vi "F8588A set & read standalone.vi"() -> ()   [LabVIEW 2020]
uses:
  0877c1e3-cff1-4e1c-ae5b-e7c7f4b59a18.vi
  eb5dc96a-a43c-4ad0-98b0-8bae309643aa.vi
  <vilib>/Analysis/NI_AALBase.lvlib
panel:
  out "time to read data (ms)":u32
  out "type A uncertainty":dbl format="%.9pV"
  out "samples":i32
  out "standard deviation":dbl format="%.9pV"
  out "mean":dbl format="%.9pV"
  in  "Initialization configuration":string="*CLS\n*RST\nDISP ON;\n*CLS\nFUNC \"DIG:VOLT\";DIG:VOLT:RANG 10.000000;\nDIG:FILT OFF;:SENS:DIG:VOLT:COUP:SIGN DCAuto;:TRIG:RESET;:TRIG:ECO 1;:ARM:LAY2:SOUR IMM;:ARM:LAY2:COUNT 1;:ARM:LAY1:COUNT 1;:ARM:LAY2:ECO 1;:ARM:LAY1:ECO 1;:ROUT:TOUT APE;:ROUT:INP:GUARD 0\nDIG:VOLT:RANG 10.000000;\n:ARM:LAY2:SOUR IMM;:ARM:LAY1:SOUR IMM;:TRIG:COUNT 101010;:TRIG:SOUR TIMER;\n:TRIG:TIMER 200E-9;\n:SENS:DIG:APER 200E-9;\nFORM PACK,2;FORM:BORD SWAP;\n:ARM:LAY1:SLOP POS;:ARM:LAY1:LEV 0.00000;:ARM:LAY1:COUP DC;\n:ARM:LAY1:DEL 1.000000E-7;\nROUT:TOUT APE;\n*CLS;"
  out "XY Graph":cluster{dbl[], dbl[]}(graph)
  out "form scale":dbl
  out "error 1":errorcluster
  out "buffer length":i32
  out "FORM?":string
  out "error 2":errorcluster
  out "read buffer":string
  # "Basic IV to test errors of F8588 communications"
  # "ASC\ndata:\n+8.407E-2\n+9.497E-2\ndecimal dot, new line as line feed (\\n),\n\nPACK,4\ndata:\nAD30 AAFF 0000 0000 8C5F 99FF 0000 0000 90E8 88FF 0000 0000\nreshape every 2nd, keep length 1, I32 little endian\n\nPACK,2\ndata:\n6CFE 2000 0000 0000 74FE 2000 0000 0000 \nreshape every 4th, keep length 1, I16 little endian\n\nPACK - nefunguje"
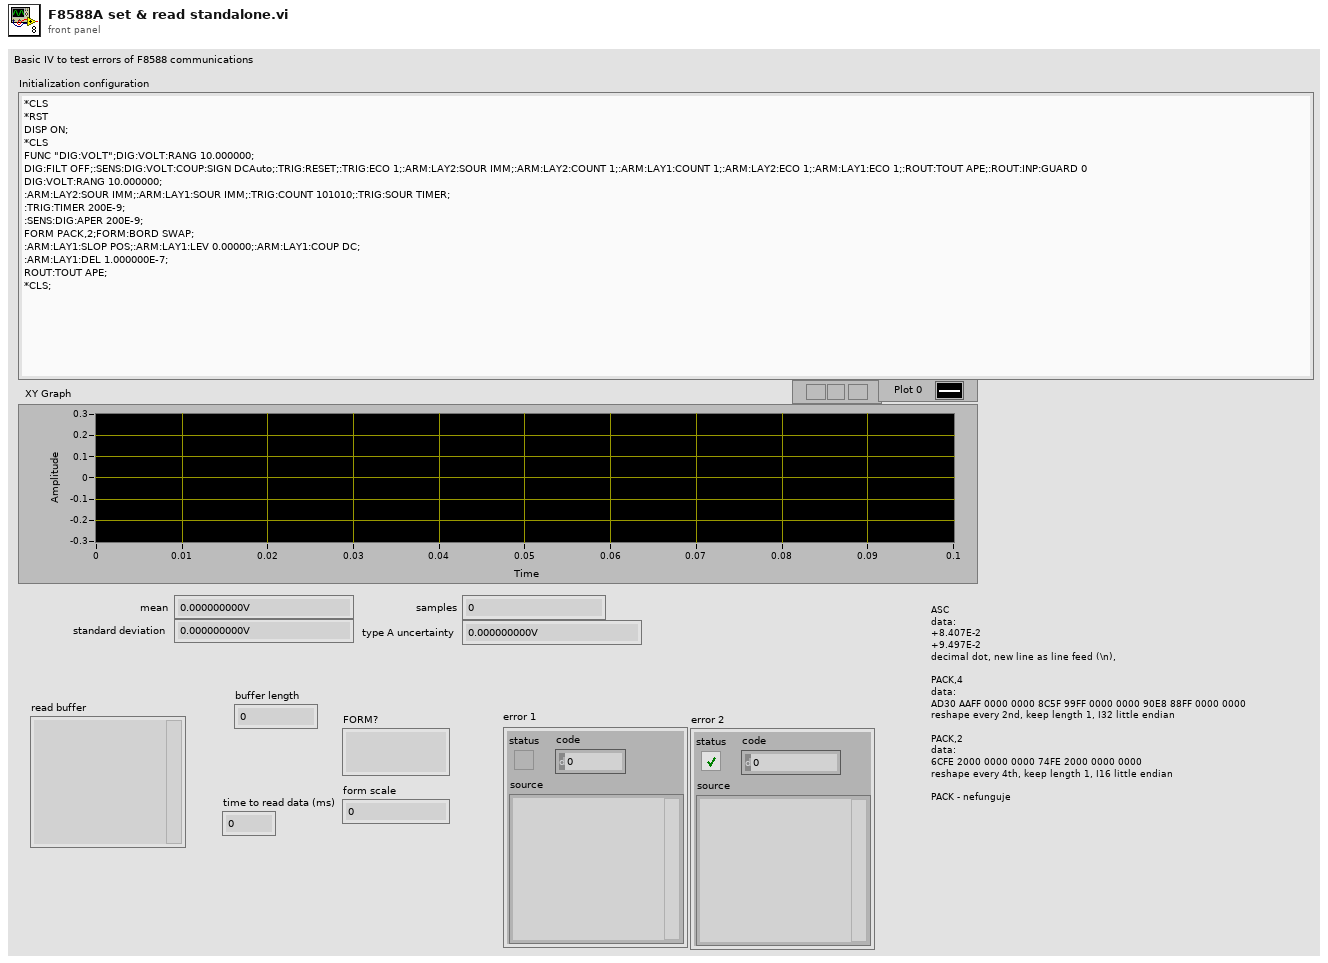
[diagram p1: front panel]
types:
  T1 = enum16{"big-endian, network order", "native, host order", "little-endian"}
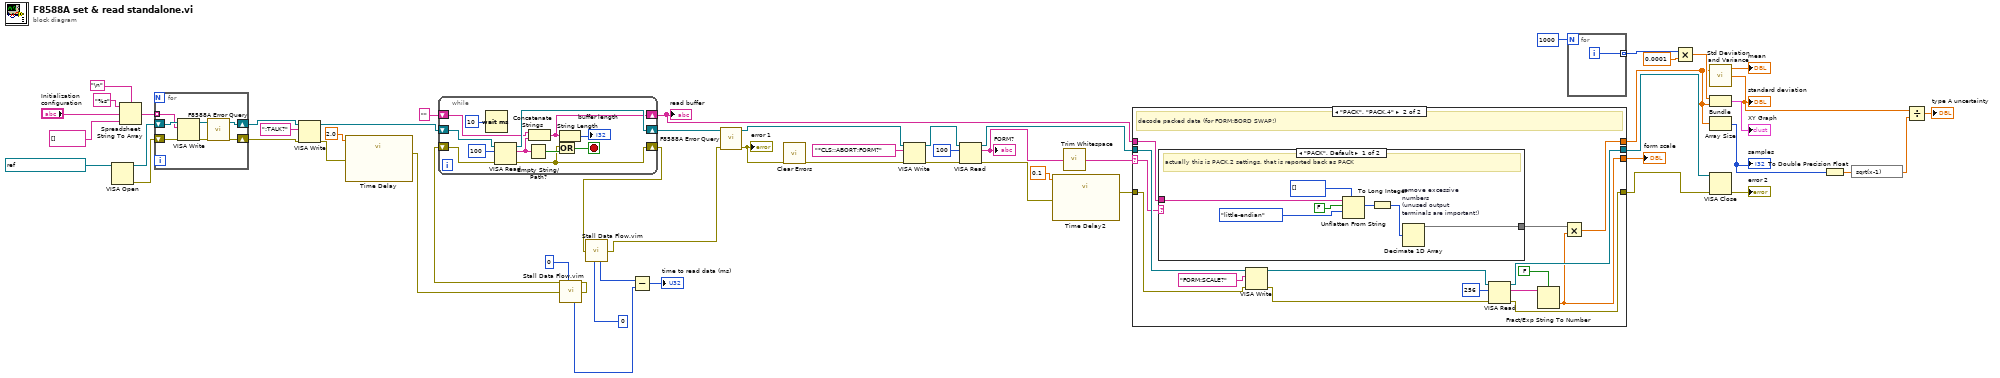
[diagram p0: block diagram]
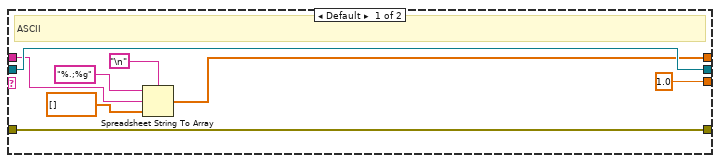
[diagram p2: hidden frame]
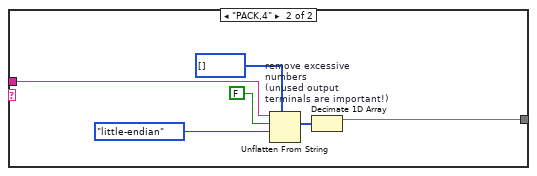
[diagram p3: hidden frame]
diagram:
  n1 = VISA Open(VISA resource name=refnum<visa-resource-name> "GPIB0::10::INSTR") -> (VISA resource name=w51:refnum<visa-resource-name>, error out=w52:errorcluster)  [unwired: 4 in]
  n2 = Spreadsheet String To Array(delimiter (Tab)="\n", format string="%s", spreadsheet string="Initialization configuration", array type (2D Dbl)=string[] []) -> (array=w46:string[])
  n3 = for {
    tunnel: w46 -> [w60] mode=indexing
    shift-right: [w58] -> w37
    shift-left: w52 -> [w62]
    shift-right: [w57] -> w38
    shift-left: w51 -> [w61]
    n4 = VISA Write(VISA resource name=w61, write buffer=w60, error in (no error)=w62) -> (VISA resource name out=w56:refnum<visa-resource-name>, error out=w59:errorcluster)  [unwired: 1 out]
    n5 = call "F8588A Error Query.vi"("error in (no error)"=w59, "VISA resource name"=w56) -> ("error out"=w58:errorcluster, "VISA resource name out"=w57:refnum<visa-resource-name>)  [unwired: 6 in, 2 out]
  }
  n6 = VISA Write(VISA resource name=w38, write buffer=":TALK?", error in (no error)=w37) -> (VISA resource name out=w35:refnum<visa-resource-name>, error out=w36:errorcluster)  [unwired: 1 out]
  n7 = call "Time Delay"("error in (no error)"=w36, "Delay Time (s)"=2.0) -> ("error out"=w4:errorcluster)  [unwired: 9 in]
  n8 = call "Stall Data Flow.vim"("value in"=w4, "milliseconds to wait"=u32 0) -> ("millisecond timer value"=w8:u32, "value out"=w3:errorcluster)
  n9 = while {
    shift-right: [w67] -> w2
    shift-left: w3 -> [w73]
    shift-right: [w72] -> w40
    shift-left: w35 -> [w71]
    shift-right: [w64] -> w25
    shift-left: "" -> [w63]
    stop <- w68 stop-if-true
    n10 = Wait (ms)(milliseconds to wait=u32 10) -> ()  [unwired: 1 out]
    n11 = VISA Read(VISA resource name=w71, byte count=u32 100, error in (no error)=w73) -> (VISA resource name out=w72:refnum<visa-resource-name>, read buffer=w70:string, error out=w67:errorcluster)  [unwired: 1 out]
    n12 = Empty String/Path?(string/path=w70) -> (empty?=w69:bool)
    n13 = Concatenate Strings(w63, w70) -> (w64:string)
    n14 = Or(x=w67, y=w69) -> (x .or. y?=w68:bool)
    n15 = String Length(string=w64) -> (length=→"buffer length":i32)
  }
  "read buffer" <- w25
  n16 = call "Stall Data Flow.vim"("value in"=w2, "milliseconds to wait"=u32 0) -> ("millisecond timer value"=w9:u32, "value out"=w1:errorcluster)
  n17 = Subtract(x=w9, y=w8) -> (x-y=→"time to read data (ms)":u32)
  n18 = call "F8588A Error Query.vi"("error in (no error)"=w1, "VISA resource name"=w40) -> ("error out"=w33:errorcluster, "VISA resource name out"=w39:refnum<visa-resource-name>)  [unwired: 6 in, 2 out]
  "error 1" <- w33
  n19 = call <vilib>:"Clear Errors.vi"("error in (no error)"=w33) -> ("error out"=w32:errorcluster)  [unwired: 5 in, 1 out]
  n20 = VISA Write(VISA resource name=w39, write buffer="*CLS;:ABORT;FORM?", error in (no error)=w32) -> (VISA resource name out=w44:refnum<visa-resource-name>, error out=w45:errorcluster)  [unwired: 1 out]
  n21 = VISA Read(VISA resource name=w44, byte count=u32 100, error in (no error)=w45) -> (VISA resource name out=w29:refnum<visa-resource-name>, read buffer=w27:string, error out=w42:errorcluster)  [unwired: 1 out]
  "FORM?" <- w27
  n22 = call "Time Delay2"("error in (no error)"=w42, "Delay Time (s)"=0.1) -> ("error out"=w6:errorcluster)  [unwired: 9 in]
  n23 = call <vilib>:"Trim Whitespace.vi"("string"=w27) -> ("trimmed string"=w26:string)  [unwired: 1 in]
  n24 = case shown="\"PACK\", \"PACK,4\"" w26 {
    selector: w26 -> [_ w85]
    tunnel: [w81 w92] -> w5
    tunnel: [w82 w91] -> w28
    tunnel: w29 -> [w82 w90]
    tunnel: w6 -> [w81 w89]
    tunnel: [1.0 w87] -> w24
    tunnel: w25 -> [w76 w86]
    tunnel: [w75 w84] -> w17
    frame Default {
      # "ASCII"
      n25 = Spreadsheet String To Array(delimiter (Tab)="\n", format string="%.;%g", spreadsheet string=w76, array type (2D Dbl)=dbl[] []) -> (array=w75:dbl[])
    }
    frame "PACK", "PACK,4" {
      # "decode packed data (for FORM:BORD SWAP!)"
      n26 = case shown="\"PACK\", Default" w85 {
        tunnel: w86 -> [w104 w110]
        tunnel: [w98 w105] -> w83
        frame "PACK", Default {
          # "actually this is PACK,2 settings, that is reported back as PACK"
          n27 = Unflatten From String(type=i16[] [], binary string=w104, data includes array or string size? (T)=FALSE, byte order (0:big-endian, network order)=T1."little-endian") -> (value=w100:i16[])  [unwired: 1 in, 2 out]
          n28 = To Long Integer(number=w100) -> (32bit integer=w99:i32[])
          n29 = Decimate 1D Array "remove excessive\nnumbers\n(unused output\nterminals are important!)"(w99) -> (w98:i32[])  [unwired: 3 out]
        }
        frame "PACK,4" {
          n30 = Unflatten From String(type=i32[] [], binary string=w110, data includes array or string size? (T)=FALSE, byte order (0:big-endian, network order)=T1."little-endian") -> (value=w106:i32[])  [unwired: 1 in, 2 out]
          n31 = Decimate 1D Array "remove excessive\nnumbers\n(unused output\nterminals are important!)"(w106) -> (w105:i32[])  [unwired: 1 out]
        }
      }
      n32 = VISA Write(VISA resource name=w90, write buffer="FORM:SCALE?", error in (no error)=w89) -> (VISA resource name out=w95:refnum<visa-resource-name>, error out=w94:errorcluster)  [unwired: 1 out]
      n33 = VISA Read(VISA resource name=w95, byte count=u32 256, error in (no error)=w94) -> (VISA resource name out=w91:refnum<visa-resource-name>, read buffer=w88:string, error out=w92:errorcluster)  [unwired: 1 out]
      n34 = Fract/Exp String To Number(use system decimal point (T)=FALSE, string=w88) -> (number=w87:dbl)  [unwired: 2 in, 1 out]
      n35 = Multiply(x=w83, y=w87) -> (x*y=w84:dbl[])
    }
  }
  "form scale" <- w24
  n36 = for {
    N: 1000 -> [_]
    tunnel: [w111] -> w22 mode=indexing
    i -> [w111]
  }
  n37 = Multiply(x=w22, y=0.0001) -> (x*y=w19:dbl[])
  n38 = call <vilib>:"Std Deviation and Variance.vi"("X"=w17) -> ("mean"=→"mean":dbl, "standard deviation"=w13:dbl)  [unwired: 1 in, 1 out]
  "standard deviation" <- w13
  n39 = Bundle(w19, "array type (2D Dbl)"=w17) -> (→"XY Graph":cluster{dbl[], "array type (2D Dbl)":dbl[]})  [unwired: 1 in]
  n40 = Array Size(array=w17) -> (size(s)=w15:i32)
  "samples" <- w15
  n41 = VISA Close(VISA resource name=w28, error in (no error)=w5) -> (error out=→"error 2":errorcluster)
  n42 = To Double Precision Float(number=w15) -> (double precision float=w16:dbl)
  n43 = expression code="sqrt(x-1)"(w16) -> (w14:dbl)
  n44 = Divide(x=w13, y=w14) -> (x/y=→"type A uncertainty":dbl)
